vi "Configure.vi"(8 "error in (no error)":errorcluster caption="错误输入（无错误）", 11 "34461A 输入":refnum<class "34461A.lvclass">) -> (0 "error out":errorcluster caption="错误输出", 3 "34461A 输出":refnum<class "34461A.lvclass">)   [LabVIEW 2020, in "34461A.lvlib" / "34461A.lvclass"]
uses:
  34461A.lvclass
  <instrlib>/Agilent 3446X Series/Agilent 3446X Series.lvlib
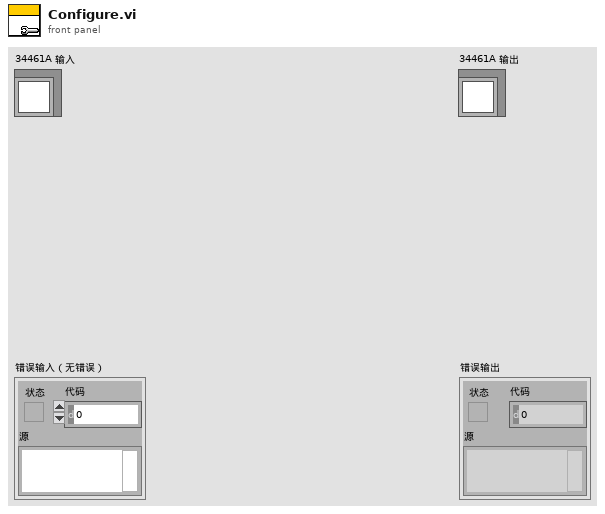
[diagram p1: front panel]
types:
  T1 = enum16{"DC Voltage", "AC Voltage", "Resistance", "DC Current", "AC Current"}
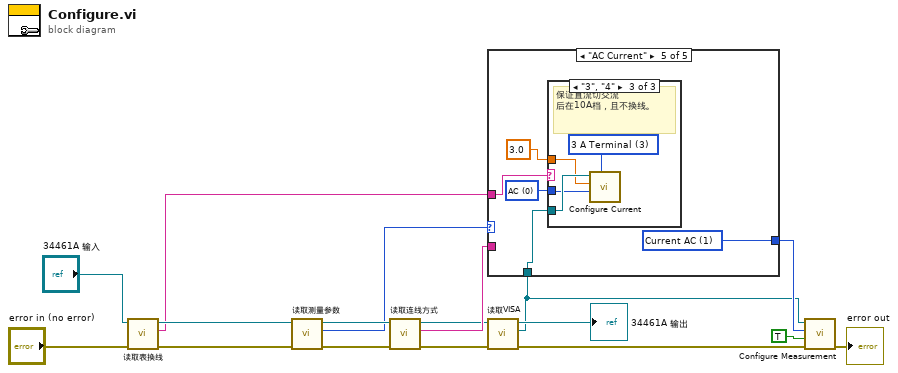
[diagram p0: block diagram]
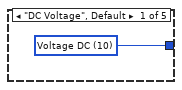
[diagram p2: hidden frame]
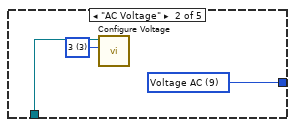
[diagram p3: hidden frame]
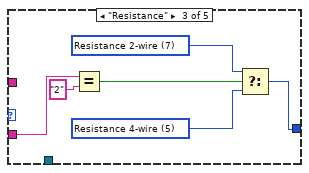
[diagram p4: hidden frame]
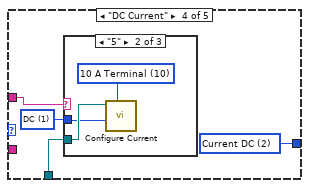
[diagram p5: hidden frame]
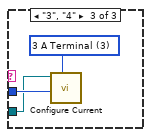
[diagram p7: hidden frame]
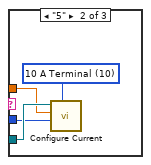
[diagram p9: hidden frame]
diagram:
  n1 = call "读取表换线.vi"("error in (no error)"="error in (no error)", "数字多用表接口输入"="34461A 输入") -> ("error out"=w10:errorcluster, "表换线"=w2:string, "数字多用表接口输出"=w11:refnum<class "34461A.lvclass">)  [unwired: 7 in]
  n2 = call "读取测量参数.vi"("error in (no error)"=w10, "数字多用表接口输入"=w11) -> ("error out"=w15:errorcluster, "测量参数"=w14:T1, "数字多用表接口输出"=w17:refnum<class "34461A.lvclass">)  [unwired: 7 in]
  n3 = call "读取连线方式.vi"("error in (no error)"=w15, "数字多用表接口输入"=w17) -> ("error out"=w12:errorcluster, "连线方式"=w16:string, "数字多用表接口输出"=w13:refnum<class "34461A.lvclass">)  [unwired: 7 in]
  n4 = call "读取VISA.vi"("error in (no error)"=w12, "数字多用表接口输入"=w13) -> ("error out"=w4:errorcluster, "VISA"=w1:refnum<visa-resource-name>, "数字多用表接口输出"=→"34461A 输出":refnum<class "34461A.lvclass">)  [unwired: 7 in]
  n5 = case shown="\"AC Current\"" w14 {
    tunnel: [w18 w21 w24 w31 w42] -> w6
    tunnel: w16 -> [_ _ w25 _ _]
    tunnel: w2 -> [_ _ _ w30 w39]
    tunnel: w1 -> [_ w20 _ w28 w40]
    frame "DC Voltage", Default {
      w18 = 10 items=["Continuity", "Current AC", "Current DC", "Diode", "Frequency", "Resistance 4-wire", "Period", "Resistance 2-wire", "Temperature", "Voltage AC", "Voltage DC", "Voltage DC Ratio", "Capacitance"] ("Measurement Function (10: Voltage DC)")
    }
    frame "AC Voltage" {
      w19 = 3 items=["3"=3, "20"=20, "200"=200] ("Voltage Bandwidth (20: 20 Hz)")
      w21 = 9 items=["Continuity", "Current AC", "Current DC", "Diode", "Frequency", "Resistance 4-wire", "Period", "Resistance 2-wire", "Temperature", "Voltage AC", "Voltage DC", "Voltage DC Ratio", "Capacitance"] ("Measurement Function (10: Voltage DC)")
      n6 = call <instrlib>:"Configure Voltage.vi"("Voltage Bandwidth (20: 20 Hz)"=w19, "VISA resource name"=w20) -> ()  [unwired: 8 in, 2 out]
    }
    frame "Resistance" {
      w22 = 5 items=["Continuity", "Current AC", "Current DC", "Diode", "Frequency", "Resistance 4-wire", "Period", "Resistance 2-wire", "Temperature", "Voltage AC", "Voltage DC", "Voltage DC Ratio", "Capacitance"] ("Measurement Function (10: Voltage DC)")
      w23 = 7 items=["Continuity", "Current AC", "Current DC", "Diode", "Frequency", "Resistance 4-wire", "Period", "Resistance 2-wire", "Temperature", "Voltage AC", "Voltage DC", "Voltage DC Ratio", "Capacitance"] ("Measurement Function (10: Voltage DC)")
      n7 = Equal?(x=w25, y="2") -> (x = y?=w27:bool)
      n8 = Select(t=w23, s=w27, f=w22) -> (s? t:f=w24:i32)
    }
    frame "DC Current" {
      w29 = 1 items=["AC", "DC"] ("Current Type (0: AC)")
      w31 = 2 items=["Continuity", "Current AC", "Current DC", "Diode", "Frequency", "Resistance 4-wire", "Period", "Resistance 2-wire", "Temperature", "Voltage AC", "Voltage DC", "Voltage DC Ratio", "Capacitance"] ("Measurement Function (10: Voltage DC)")
      n9 = case shown="\"5\"" w30 {
        tunnel: w29 -> [_ w32 w36]
        tunnel: w28 -> [_ w33 w35]
        frame "0", Default {
        }
        frame "5" {
          w34 = 10 items=["3 A Terminal"=3, "10 A Terminal"=10] ("Terminal Type (3: 3 A Terminal)")
          n10 = call <instrlib>:"Configure Current.vi"("Terminal Type (3: 3 A Terminal)"=w34, "Current Type (0: AC)"=w32, "VISA resource name"=w33) -> ()  [unwired: 7 in, 2 out]
        }
        frame "3", "4" {
          w37 = 3 items=["3 A Terminal"=3, "10 A Terminal"=10] ("Terminal Type (3: 3 A Terminal)")
          n11 = call <instrlib>:"Configure Current.vi"("Terminal Type (3: 3 A Terminal)"=w37, "Current Type (0: AC)"=w36, "VISA resource name"=w35) -> ()  [unwired: 7 in, 2 out]
        }
      }
    }
    frame "AC Current" {
      w38 = 3.0 items=["3"=3.0, "20"=20.0, "200"=200.0] ("Current Bandwidth (20 Hz)")
      w41 = 0 items=["AC", "DC"] ("Current Type (0: AC)")
      w42 = 1 items=["Continuity", "Current AC", "Current DC", "Diode", "Frequency", "Resistance 4-wire", "Period", "Resistance 2-wire", "Temperature", "Voltage AC", "Voltage DC", "Voltage DC Ratio", "Capacitance"] ("Measurement Function (10: Voltage DC)")
      n12 = case shown="\"3\", \"4\"" w39 {
        tunnel: w41 -> [_ w44 w48]
        tunnel: w40 -> [_ w45 w49]
        tunnel: w38 -> [_ w43 w47]
        frame "0", Default {
        }
        frame "5" {
          w46 = 10 items=["3 A Terminal"=3, "10 A Terminal"=10] ("Terminal Type (3: 3 A Terminal)")
          n13 = call <instrlib>:"Configure Current.vi"("Terminal Type (3: 3 A Terminal)"=w46, "Current Type (0: AC)"=w44, "Current Bandwidth (20 Hz)"=w43, "VISA resource name"=w45) -> ()  [unwired: 6 in, 2 out]
        }
        frame "3", "4" {
          w50 = 3 items=["3 A Terminal"=3, "10 A Terminal"=10] ("Terminal Type (3: 3 A Terminal)")
          # "保证直流切交流\n后在10A档，且不换线。"
          n14 = call <instrlib>:"Configure Current.vi"("Terminal Type (3: 3 A Terminal)"=w50, "Current Type (0: AC)"=w48, "Current Bandwidth (20 Hz)"=w47, "VISA resource name"=w49) -> ()  [unwired: 6 in, 2 out]
        }
      }
    }
  }
  n15 = call <instrlib>:"Configure Measurement.vi"("error in (no error)"=w4, "Auto Range (T: Enable)"=TRUE ("Enable Auto Range (T: Enable)"), "Measurement Function (10: Voltage DC)"=w6, "VISA resource name"=w1) -> ("error out"=→"error out":errorcluster)  [unwired: 6 in, 1 out]
